vi "Read SSH.vi"(8 "Error In":errorcluster, 11 "Agent In":refnum<class "Agent.lvclass">) -> (0 "Error Out":errorcluster, 2 "SSH":refnum<class "SSH.lvclass">, 3 "Agent Out":refnum<class "Agent.lvclass">)   [LabVIEW 2021, in "Field_RnD_Services_LIBSSH2_Toolkit.lvlib" / "Agent.lvclass"]
doc: "Gets the SSH context that created this Agent object."
uses:
  220524-VNA RP FLAT.llb/Agent.lvclass
  220524-VNA RP FLAT.llb/SSH.lvclass
  220524-VNA RP FLAT.llb/Agent.lvclass/Agent.ctl
  220524-VNA RP FLAT.llb/Session.lvclass
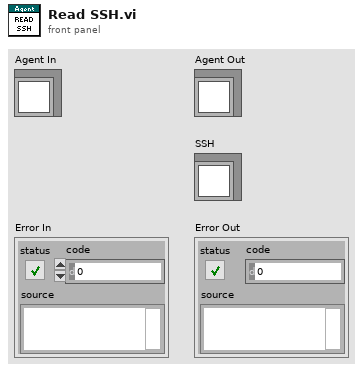
[diagram p1: front panel]
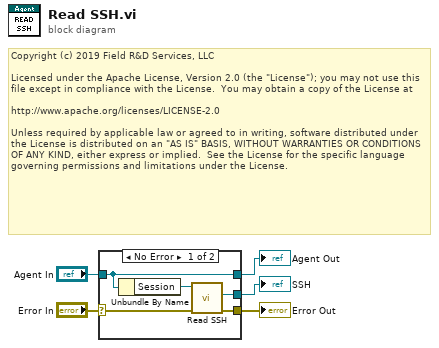
[diagram p0: block diagram]
diagram:
  # "Copyright (c) 2019 Field R&D Services, LLC\n\nLicensed under the Apache License, Version 2.0 (the \"License\"); you may not use this file except in compliance with the License.  You may obtain a copy of the License at\n\nhttp://www.apache.org/licenses/LICENSE-2.0\n\nUnless required by applicable law or agreed to in writing, software distributed under the License is distributed on an \"AS IS\" BASIS, WITHOUT WARRANTIES OR CONDITIONS OF ANY KIND, either express or implied.  See the License for the specific language governing permissions and limitations under the License."
  n1 = case shown="No Error" "Error In" {
    selector: "Error In" -> [w8 w11]
    tunnel: "Agent In" -> [w10 w12]
    tunnel: [w10 w12] -> w1
    tunnel: [w6 w11] -> w4
    tunnel: [w7 _] -> w3
    frame No Error {
      n2 = Unbundle By Name(w10) -> ("Session"=w9:refnum<class "Session.lvclass">)
      n3 = call "Read SSH.vi"("Error In"=w8, "Session In"=w9) -> ("Erorr Out"=w6:errorcluster, "SSH"=w7:refnum<class "SSH.lvclass">)  [unwired: 7 in, 1 out]
    }
    frame Error {
    }
  }
  "Error Out" <- w4
  "SSH" <- w3
  "Agent Out" <- w1
